vi "STRING_POT_CAL.vi"(8 "error in (no error)":errorcluster, 11 "string_pot_slope_IN":dbl=51.35 format="%.2f") -> (0 "error out":errorcluster, 3 "string_pot_slope_OUT":dbl=51.35 format="%.2f")   [LabVIEW 2016]
uses:
  ad interface/Global_SIM_switch.vi
panel:
  out "Distance(ft)":dbl format="%.2f"
  in  "stop":bool
  in  "start":bool
  # "STRING POTENTIOMETER CALIBRATION"
  # "Hold string pot wire at 5' above the string pot body.\nPress start."
  # "Slowly lower the string pot wire.\nPress Stop when t he string pot wire is fully retracted."
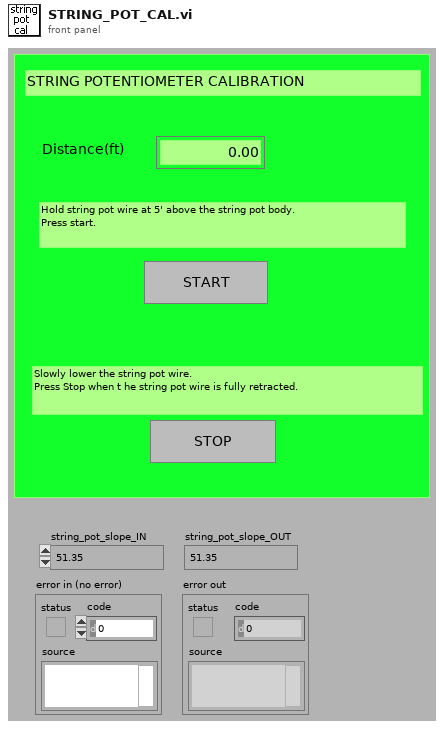
[diagram p1: front panel]
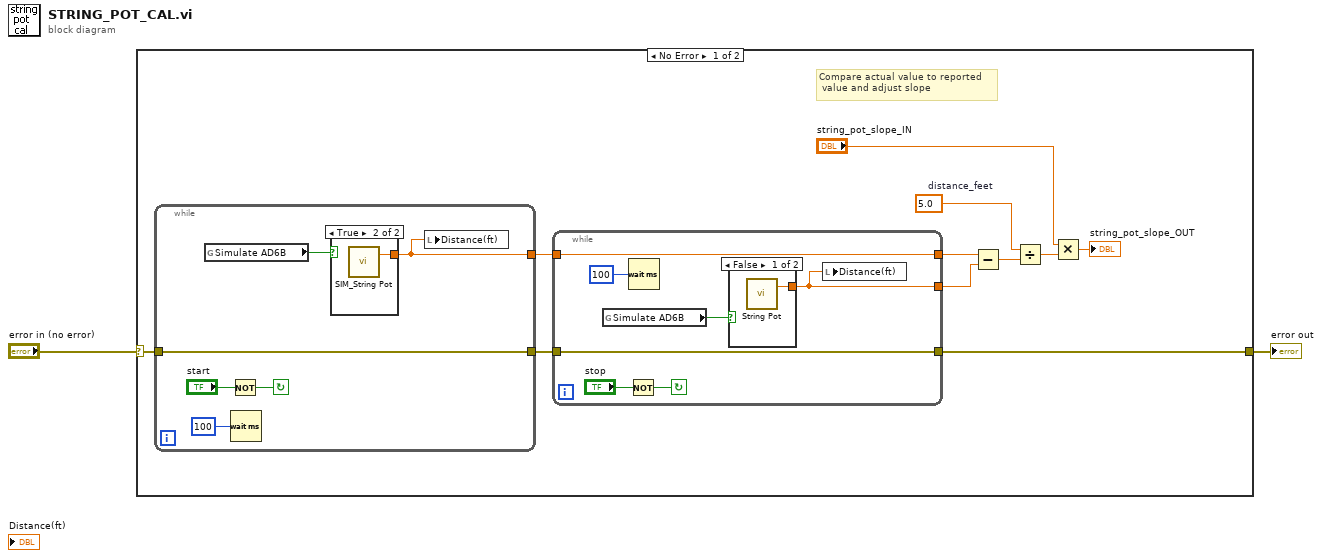
[diagram p0: block diagram]
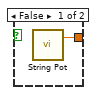
[diagram p2: hidden frame]
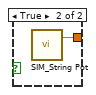
[diagram p3: hidden frame]
diagram:
  n1 = case shown="No Error" "error in (no error)" {
    selector: "error in (no error)" -> [w13 w31]
    tunnel: [w11 w31] -> w2
    frame No Error {
      w10 = 5.0  # distance_feet
      # "Compare actual value to reported\n value and adjust slope"
      n2 = while {
        tunnel: [w14] -> w7
        tunnel: [w17] -> w12
        tunnel: w13 -> [w17]
        stop <- w18 continue-if-true
        n3 = global read "Global_SIM_switch.vi" "Simulate AD6B"() -> (w16:bool)
        n4 = Not(x="start") -> (.not. x?=w18:bool)
        n5 = Wait (ms)(milliseconds to wait=u32 100) -> ()  [unwired: 1 out]
        n6 = case shown="True" w16 {
          tunnel: [w20 w21] -> w14
          frame False {
            n7 = call "String Pot.vi"() -> ("Distance (in)"=w20:dbl)  [unwired: 3 in]
          }
          frame True {
            n8 = call "SIM_String Pot.vi"() -> ("Distance (in)"=w21:dbl)  [unwired: 3 in]
          }
        }
        n9 = local write "Distance(ft)"(w14) -> ()
      }
      n10 = while {
        tunnel: w7 -> [w24]
        tunnel: [w22] -> w4
        tunnel: [w24] -> w3
        tunnel: w12 -> [w25]
        tunnel: [w25] -> w11
        stop <- w28 continue-if-true
        n11 = global read "Global_SIM_switch.vi" "Simulate AD6B"() -> (w26:bool)
        n12 = Not(x="stop") -> (.not. x?=w28:bool)
        n13 = Wait (ms)(milliseconds to wait=u32 100) -> ()  [unwired: 1 out]
        n14 = case shown="False" w26 {
          tunnel: [w29 w30] -> w22
          frame False {
            n15 = call "String Pot.vi"() -> ("Distance (in)"=w29:dbl)  [unwired: 3 in]
          }
          frame True {
            n16 = call "SIM_String Pot.vi"() -> ("Distance (in)"=w30:dbl)  [unwired: 3 in]
          }
        }
        n17 = local write "Distance(ft)"(w22) -> ()
      }
      n18 = Subtract(x=w3, y=w4) -> (x-y=w6:dbl)
      n19 = Divide(x=w10, y=w6) -> (x/y=w5:dbl)
      n20 = Multiply(x="string_pot_slope_IN", y=w5) -> (x*y=→"string_pot_slope_OUT":dbl)
    }
    frame Error {
    }
  }
  "error out" <- w2
